vi "ScanEngine.vi"(7 "Action":T1, 8 "Metric Control":T2, 11 "Abberation Cluster":T4 {"Modes"."Amplititude" step=0.05}) -> (0 "Metric Image":sgl[][](array[numeric]), 2 "Metric Result":dbl)   [LabVIEW 2014]
uses:
  DMControl_STED.ctl
  MetricControl.ctl
  Scan Metric.ctl
  ScanEngineState.ctl
panel:
  out "created new?":bool
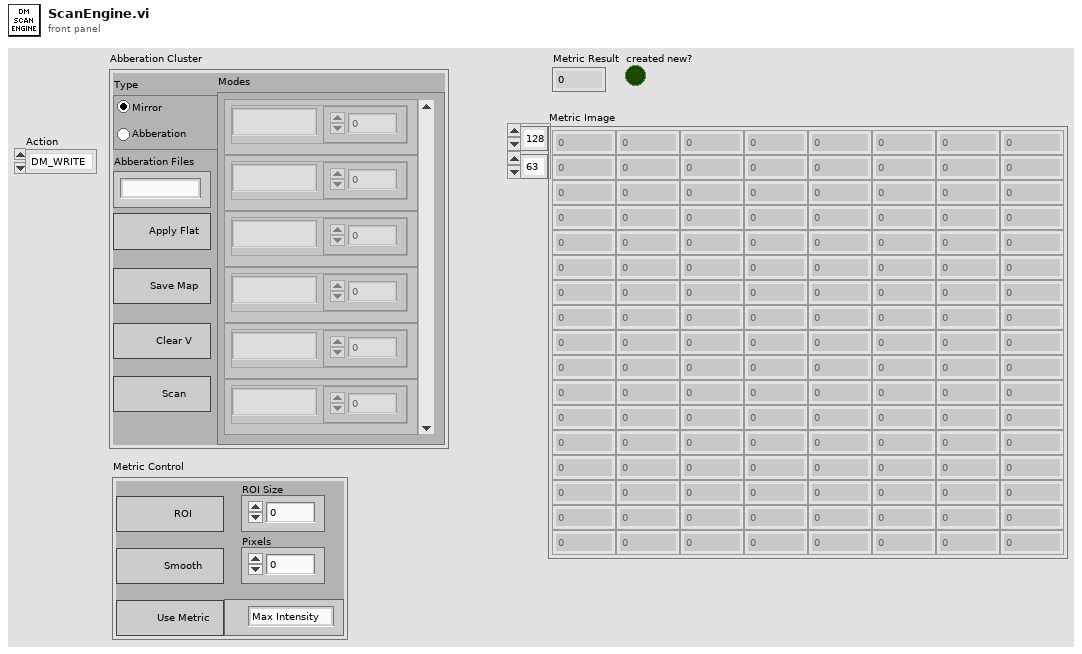
[diagram p1: front panel]
types:
  T1 = typedef "ScanEngineState.ctl" = enum16{"DM_WRITE", "IMAGE", ""}
  T2 = typedef "MetricControl.ctl" = cluster{"Use Metric":bool, "DM Metric":T3, "Smooth":bool, "Pixels":dbl, "ROI":bool, "ROI Size":dbl}
  T3 = typedef "Scan Metric.ctl" = enum16{"Max Intensity", "No Zero Mean", "Threshold"}
  T4 = typedef "DMControl_STED.ctl" = cluster{"Type":enum32{"Mirror", "Abberation"}, "Modes":cluster{"Mode":string, "Amplititude":dbl}[], "Apply Flat":bool, "Save Map":bool, "Clear Voltage":bool, "Abberation Files":u16, "Scan ":bool}
  T5 = typedef "AbberationControl.ctl" = cluster{"Abberations":dbl[][], "Modes":i32[], "Abberations ID":string[], "Abberation Files":path[]}
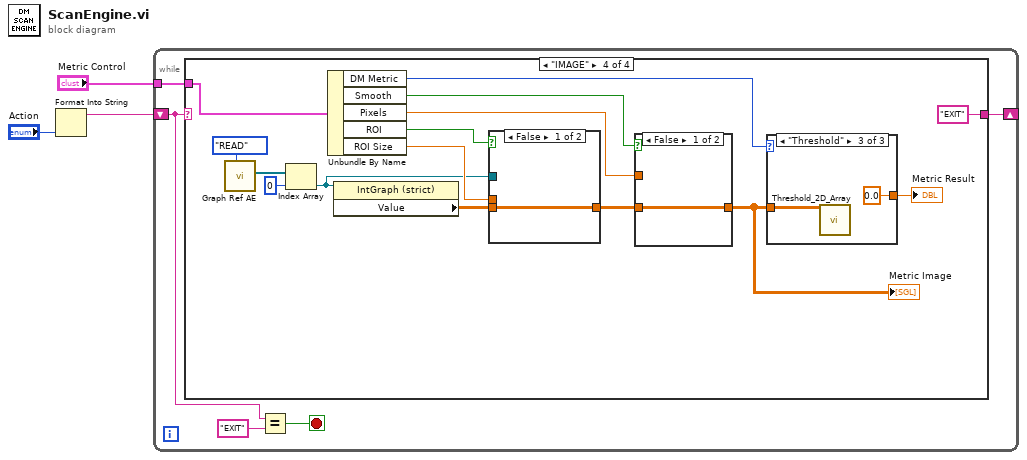
[diagram p0: block diagram]
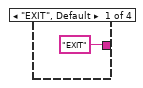
[diagram p2: hidden frame]
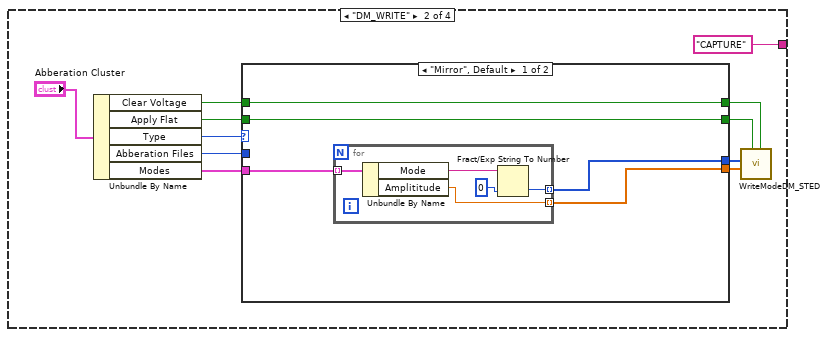
[diagram p3: hidden frame]
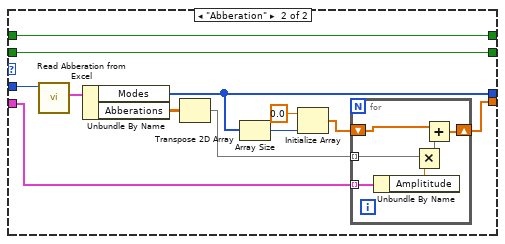
[diagram p4: hidden frame]
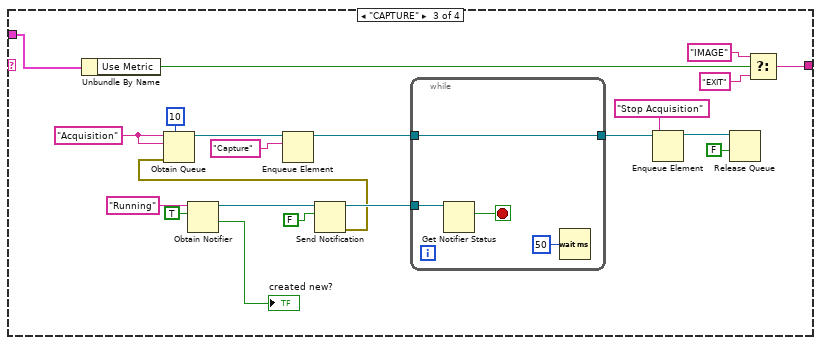
[diagram p5: hidden frame]
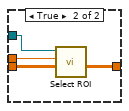
[diagram p6: hidden frame]
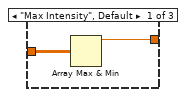
[diagram p7: hidden frame]
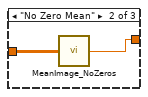
[diagram p8: hidden frame]
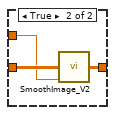
[diagram p9: hidden frame]
diagram:
  n1 = Format Into String("Action") -> (resulting string=w1:string)  [unwired: 3 in, 1 out]
  n2 = while {
    shift-right: [w8] -> _
    shift-left: w1 -> [w7]
    tunnel: "Metric Control" -> [w4]
    stop <- w5 stop-if-true
    n3 = case shown="\"IMAGE\"" w7 {
      tunnel: ["EXIT" "CAPTURE" w66 "EXIT"] -> w8
      tunnel: w4 -> [_ _ w57 w85]
      frame "EXIT", Default {
      }
      frame "DM_WRITE" {
        n4 = Unbundle By Name("Abberation Cluster") -> ("Clear Voltage"=w12:bool, "Apply Flat"=w14:bool, "Type"=w20:enum32{"Mirror", "Abberation"}, "Abberation Files"=w19:u16, "Modes"=w17:cluster{"Mode":string, "Amplititude":dbl}[])
        n5 = case shown="\"Mirror\", Default" w20 {
          tunnel: w19 -> [_ w42]
          tunnel: [w21 w36] -> w18
          tunnel: w17 -> [w23 w39]
          tunnel: [w22 w33] -> w16
          tunnel: [w24 w32] -> w15
          tunnel: w14 -> [w24 w32]
          tunnel: [w25 w31] -> w13
          tunnel: w12 -> [w25 w31]
          frame "Mirror", Default {
            n6 = for {
              tunnel: w23 -> [w30] mode=indexing
              tunnel: [w27] -> w22 mode=indexing
              tunnel: [w26] -> w21 mode=indexing
              n7 = Unbundle By Name(w30) -> ("Mode"=w28:string, "Amplititude"=w27:dbl)
              n8 = Fract/Exp String To Number(string=w28, default (0 dbl)=0) -> (number=w26:i32)  [unwired: 2 in, 1 out]
            }
          }
          frame "Abberation" {
            n9 = call "Read Abberation from Excel.vi"("Ring"=w42) -> ("output cluster"=w41:T5)  [unwired: 8 in]
            n10 = Unbundle By Name(w41) -> ("Modes"=w36:i32[], "Abberations"=w40:dbl[][])
            n11 = Transpose 2D Array(2D array=w40) -> (transposed array=w35:dbl[][])
            n12 = Array Size(array=w36) -> (size(s)=w38:i32)
            n13 = Initialize Array(0.0 ("element"), w38) -> (w34:dbl[])
            n14 = for {
              tunnel: w39 -> [w48] mode=indexing
              tunnel: w35 -> [w47] mode=indexing
              shift-right: [w43] -> w33
              shift-left: w34 -> [w45]
              n15 = Unbundle By Name(w48) -> ("Amplititude"=w46:dbl)
              n16 = Multiply(x=w47, y=w46) -> (x*y=w44:dbl[])
              n17 = Add(x=w45, y=w44) -> (x+y=w43:dbl[])
            }
          }
        }
        n18 = call "WriteModeDM_STED.vi"("ClearV"=w13, "Flat On"=w15, "Amplitudes"=w16, "Modes"=w18) -> ()  [unwired: 6 in, 2 out]
      }
      frame "CAPTURE" {
        w63 = "Acquisition" ("name (unnamed)")
        n19 = Unbundle By Name(w57) -> ("Use Metric"=w56:bool)
        n20 = Obtain Notifier(name (unnamed)="Running", notification data type=TRUE) -> (notifier out=w58:refnum<notifier>, created new?=→"created new?":bool)  [unwired: 2 in, 1 out]
        n21 = Send Notification(notification=FALSE, notifier=w58) -> (notifier out=w67:refnum<notifier>, error out=w50:errorcluster)  [unwired: 1 in]
        n22 = Obtain Queue(max queue size (-1, unlimited)=10, name (unnamed)=w63, element data type=w63, error in (no error)=w50) -> (queue out=w61:refnum<queue>)  [unwired: 1 in, 2 out]
        n23 = Enqueue Element(queue=w61, element="Capture") -> (queue out=w53:refnum<queue>)  [unwired: 2 in, 2 out]
        n24 = while {
          tunnel: w67 -> [w73]
          tunnel: w53 -> [w70]
          tunnel: [w70] -> w54
          stop <- w72 stop-if-true
          n25 = Get Notifier Status(notifier=w73) -> (current notification=w72:bool)  [unwired: 1 in, 4 out]
          n26 = Wait (ms)(milliseconds to wait=u32 50) -> ()  [unwired: 1 out]
        }
        n27 = Enqueue Element(queue=w54, element="Stop Acquisition") -> (queue out=w52:refnum<queue>)  [unwired: 2 in, 2 out]
        n28 = Release Queue(queue=w52, force destroy? (F)=FALSE) -> ()  [unwired: 1 in, 3 out]
        n29 = Select(t="IMAGE", s=w56, f="EXIT") -> (s? t:f=w66:string)
      }
      frame "IMAGE" {
        n30 = call "Graph Ref AE.vi"("Action"=enum16{"READ", "WRITE"}."READ") -> ("Graph Ref Out"=w80:refnum<vi>[])  [unwired: 10 in]
        n31 = Index Array(array=w80, index=0) -> (element=w74:refnum<vi>)
        n32 = Unbundle By Name(w85) -> ("DM Metric"=w84:T3, "Smooth"=w82:bool, "Pixels"=w83:dbl, "ROI"=w78:bool, "ROI Size"=w75:dbl)
        n33 = property class="IntGraph (strict)"(reference=w74) -> ("Value"=w76:sgl[][])  [unwired: 1 in, 2 out]
        n34 = case shown="False" w78 {
          tunnel: w76 -> [w89 w93]
          tunnel: [w89 w92] -> w77
          tunnel: w75 -> [_ w91]
          tunnel: w74 -> [_ w90]
          frame False {
          }
          frame True {
            n35 = call "Select ROI.vi"("Array In"=w93, "ROI Size"=w91, "IntensityGraph in"=w90) -> ("ROI"=w92:sgl[][])  [unwired: 8 in]
          }
        }
        n36 = case shown="False" w82 {
          tunnel: w77 -> [w100 w103]
          tunnel: [w100 w102] -> w88
          tunnel: w83 -> [_ w101]
          frame False {
          }
          frame True {
            n37 = call "SmoothImage_V2.vi"("Image IN"=w103, "Sigma (Radius)"=w101) -> ("Smoothed Image"=w102:sgl[][])  [unwired: 13 in]
          }
        }
        "Metric Image" <- w88
        n38 = case shown="\"Threshold\"" w84 {
          tunnel: w88 -> [w95 w97 w99]
          tunnel: [w94 w96 0.0 ("No Zero Mean")] -> w86
          frame "Max Intensity", Default {
            n39 = Array Max & Min(array=w95) -> (max value=w94:sgl)  [unwired: 3 out]
          }
          frame "No Zero Mean" {
            n40 = call "MeanImage_NoZeros.vi"("Image IN"=w97) -> ("No Zero Mean"=w96:dbl)  [unwired: 14 in]
          }
          frame "Threshold" {
            n41 = call "Threshold_2D_Array.vi"("2D Array IN"=w99) -> ()  [unwired: 14 in, 1 out]
          }
        }
        "Metric Result" <- w86
      }
    }
    n42 = Equal?(x=w7, y="EXIT") -> (x = y?=w5:bool)
  }
